vi "Set Initialization Data - Acq Cam.vi"(8 "error in":errorcluster, 11 "UI Cam Basler in":refnum<class "UI Cam Basler.lvclass">) -> (0 "error out":errorcluster, 3 "UI Cam Basler out":refnum<class "UI Cam Basler.lvclass">)   [LabVIEW 2023, in "UI Cam Basler.lvclass"]
doc: "Sets the initialization data of a statically linked subWorker."
uses:
  UI Cam Basler.lvclass
  Acq Cam Basler/Initialization Data.ctl
  Parsed Data Acquisition.ctl
  Data Image.ctl
  <vilib>/vision/Image Controls.llb/IMAQ Image.ctl
  <vilib>/addons/_Workers/Library/Classes/Message Queue/Message Queue.lvclass
  UI Cam Basler.lvclass/UI Cam Basler.ctl
  Acq Cam Basler/Acq Cam Basler.lvclass
  C:/Program Files (x86)/National Instruments/LabVIEW 2023/vi.lib/addons/_Workers/Library/Classes/Worker/Worker.lvclass
  <vilib>/addons/_Workers/Library/Classes/Worker/Worker.lvclass
  C:/Program Files (x86)/National Instruments/LabVIEW 2023/vi.lib/addons/_Workers/Library/Classes/Workers Object/Workers Object.lvclass
  C:/Users/flepetit/Desktop/MDI-with-Labview-Workers/Workers/UI Cam Basler/UI Cam Basler.lvclass
  C:/Program Files (x86)/National Instruments/LabVIEW 2023/vi.lib/addons/_Workers/Library/Classes/Message Queue/Message Queue.lvclass
  C:/Users/flepetit/Desktop/MDI-with-Labview-Workers/Workers/Acq Cam Basler/Acq Cam Basler.lvclass
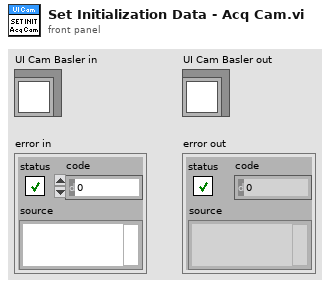
[diagram p1: front panel]
types:
  T1 = typedef "Acq Cam Basler.lvclass/Initialization Data.ctl" = cluster{"String":string, "Parsed Data Acquisition":T2, "Data Display":refnum<notifier>, "UI Cam Queue":refnum<class "Message Queue.lvclass">}
  T2 = typedef "UI Cam Basler.lvclass/Parsed Data Acquisition.ctl" = cluster{"Config Acquisition":cluster{"Camera name":string, "Gain":dbl, "Shutter(us)":dbl, "ROI":bool, "ROI coor":T3, "Palette":u32, "ModelName":string}}
  T3 = typedef "IMAQ Rectangle" = cluster{"Left":i32, "Top":i32, "Right":i32, "Bottom":i32, "Rotation":dbl}
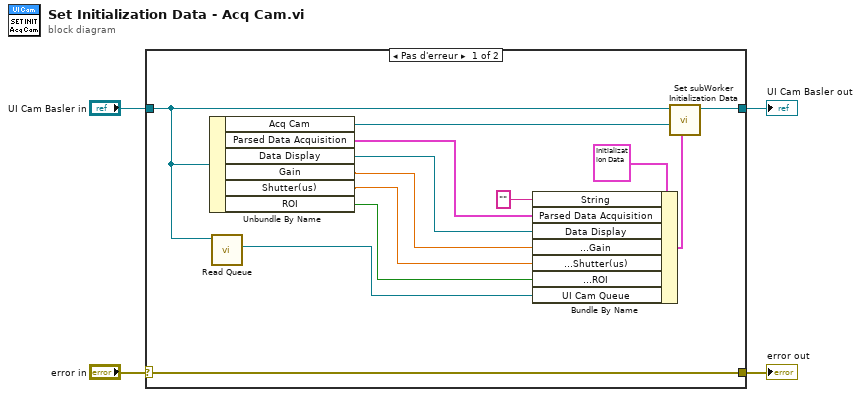
[diagram p0: block diagram]
diagram:
  n1 = case shown="Pas d'erreur" "error in" {
    selector: "error in" -> [w17 w19]
    tunnel: [w17 w19] -> w3
    tunnel: [w15 w18] -> w2
    tunnel: "UI Cam Basler in" -> [w6 w18]
    frame No Error {
      n2 = Unbundle By Name(w6) -> ("Acq Cam"=w16:refnum<class "Acq Cam Basler.lvclass">, "Parsed Data Acquisition"=w11:T2, "Data Display"=w10:refnum<notifier>, "Gain"=w9:dbl, "Shutter(us)"=w8:dbl, "ROI"=w7:bool)
      n3 = call <vilib>:"Read Queue.vi"("Worker"=w6) -> ("Message Queue out"=w5:refnum<class "Message Queue.lvclass">)  [unwired: 9 in, 1 out]
      n4 = Bundle By Name(cluster=T1 {"String"="", "Parsed Data Acquisition"={"Config Acquisition"={"Camera name"="", "Gain"=0.0, "Shutter(us)"=0.0, "ROI"=FALSE, "ROI coor"={"Left"=0, "Top"=0, "Right"=0, "Bottom"=0, "Rotation"=0.0}, "Palette"=5, "ModelName"=""}}, "Data Display"=refnum, "UI Cam Queue"=refnum} ("Initialization Data"), "String"="" ("Placeholder"), "Parsed Data Acquisition"=w11, "Data Display"=w10, "Parsed Data Acquisition.Config Acquisition.Gain"=w9, "Parsed Data Acquisition.Config Acquisition.Shutter(us)"=w8, "Parsed Data Acquisition.Config Acquisition.ROI"=w7, "UI Cam Queue"=w5) -> (w13:T1)
      n5 = call-dynamic "Set subWorker Initialization Data.vi"("Initialization Data"=w13, "subWorker"=w16, "Worker"=w6) -> ("Worker out"=w15:refnum<class "UI Cam Basler.lvclass">)  [unwired: 8 in]
    }
    frame Error {
    }
  }
  "error out" <- w3
  "UI Cam Basler out" <- w2
